vi "Examen.vi"() -> ()   [LabVIEW 2020]
uses:
  <vilib>/numeric/Random Number (Range) DBL.vi
panel:
  out "Veces que han superado el valor máximo":dbl
  out "Boton 2":bool=TRUE
  out "Dentro del rango":bool
  out "Histerísis":bool=TRUE
  out "Valor actual de EMA":dbl=70.07790415905662
  out "Valor actual de Señal Original":dbl=51.269109973451336
  out "Gráfica de datos":dbl[][](graph)=[[51.269109973451336, 70.07790415905662]]
  in  "Boton":bool
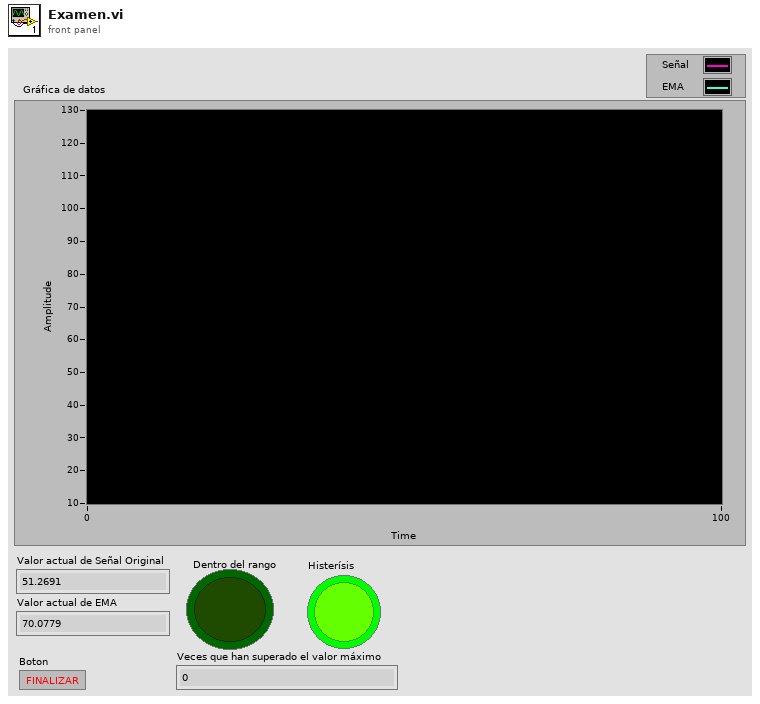
[diagram p1: front panel]
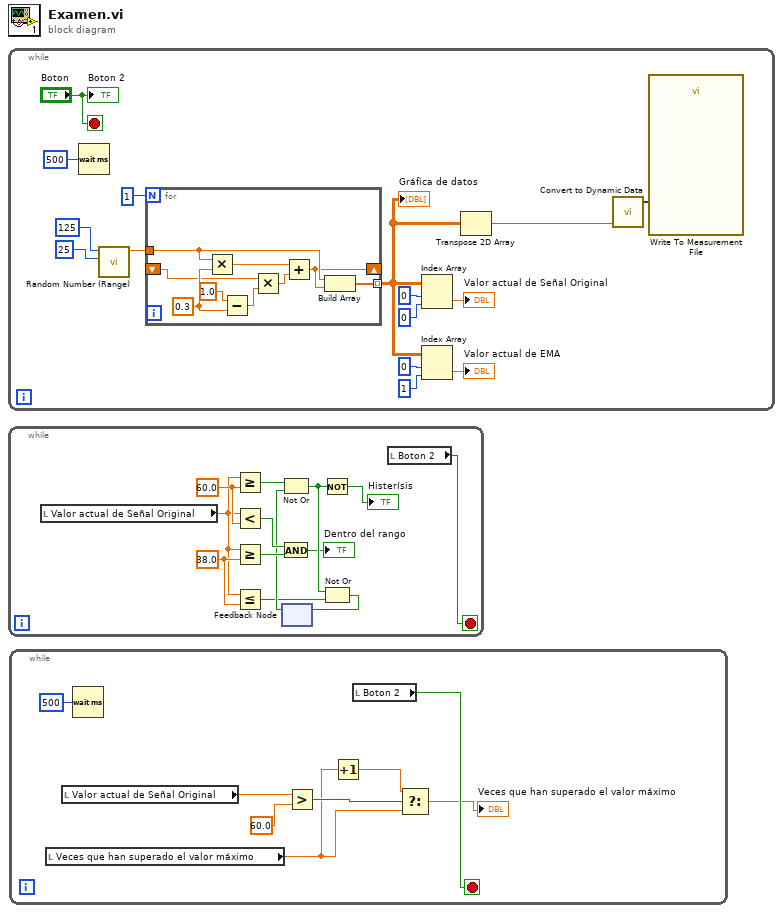
[diagram p0: block diagram]
diagram:
  n1 = while {
    stop <- "Boton" stop-if-true
    n2 = Wait (ms)(milliseconds to wait=u32 500) -> ()  [unwired: 1 out]
    n3 = call-poly <vilib>:"Random Number (Range).vi"("lower bound (0)"=u64 25, "upper bound (100)"=u64 125) -> ("number"=w10:dbl)  [unwired: 9 in]
    n4 = for {
      N: 1 -> [_]
      tunnel: w10 -> [w18]
      shift-right: [w17] -> _
      shift-left: _ -> [w19]
      tunnel: [w16] -> w3 mode=indexing
      w21 = 0.3 ("y")
      n5 = Multiply(x=w18, y=w21) -> (x*y=w24:dbl)
      n6 = Subtract(x=1.0, y=w21) -> (x-y=w23:dbl)
      n7 = Multiply(x=w19, y=w23) -> (x*y=w20:dbl)
      n8 = Add(x=w24, y=w20) -> (x+y=w17:dbl)
      n9 = Build Array(w18, w17) -> (w16:dbl[])
    }
    "Gráfica de datos" <- w3
    n10 = Index Array(array=w3, index (row)=0 ("disabled index (row)"), index (col)=0 ("disabled index (col)")) -> (element=→"Valor actual de Señal Original":dbl)
    n11 = Index Array(array=w3, index (row)=0 ("disabled index (row)"), index (col)=1 ("disabled index (col)")) -> (element=→"Valor actual de EMA":dbl)
    n12 = Transpose 2D Array(2D array=w3) -> (transposed array=w2:dbl[][])
    n13 = call "Convert to Dynamic Data"("2D Array"=w2) -> ("Dynamic Data Type"=w1:dynamicdata)  [unwired: 3 in]
    n14 = call "Write To Measurement File"("Signals"=w1) -> ()  [unwired: 16 in, 3 out]
    "Boton 2" <- "Boton"
  }
  n15 = while {
    stop <- w27 stop-if-true
    w34 = 38.0 ("MIN")
    w36 = 60.0 ("MAX")
    n16 = local read "Valor actual de Señal Original"() -> (w26:dbl)
    n17 = Greater Or Equal?(x=w26, y=w36) -> (x >= y?=w33:bool)
    n18 = Less?(x=w26, y=w36) -> (x < y?=w37:bool)
    n19 = Greater Or Equal?(x=w26, y=w34) -> (x >= y?=w35:bool)
    n20 = Less Or Equal?(x=w26, y=w34) -> (x <= y?=w30:bool)
    n21 = And(x=w37, y=w35) -> (x .and. y?=→"Dentro del rango":bool)
    n22 = feedback #1() -> (w31:bool)  [unwired: 1 in]
    n23 = Not Or(1:w31, 2:w33) -> (0:w28:bool)
    n24 = Not(x=w28) -> (.not. x?=→"Histerísis":bool)
    n25 = Not Or(1:w30, 2:w28) -> (0:w32:bool)
    n26 = feedback-in #1(w32) -> ()
    n27 = local read "Boton 2"() -> (w27:bool)
  }
  n28 = while {
    stop <- w45 stop-if-true
    n29 = local read "Veces que han superado el valor máximo"() -> (w41:dbl)
    n30 = local read "Valor actual de Señal Original"() -> (w42:dbl)
    n31 = Wait (ms)(milliseconds to wait=u32 500) -> ()  [unwired: 1 out]
    n32 = Greater?(x=w42, y=60.0) -> (0:w44:bool)
    n33 = Increment(x=w41) -> (x+1=w40:dbl)
    n34 = local read "Boton 2"() -> (w45:bool)
    n35 = Select(t=w40, s=w44, f=w41) -> (s? t:f=→"Veces que han superado el valor máximo":dbl)
  }
